vi "Digital Write 1 Channel.vi"(8 "error constant":errorcluster, 9 "Value":bool=TRUE, 10 "Channel":i32, 11 "NI-DAQ.lvclass":refnum<class "NI-DAQ.lvclass">) -> (0 "error IO":errorcluster, 3 "NI-DAQ.lvclass 2":refnum<class "NI-DAQ.lvclass">)   [LabVIEW 2019, in "NI-DAQ.lvclass"]
uses:
  NI-DAQ.lvclass
  NI-DAQ.lvclass/NI-DAQ.ctl
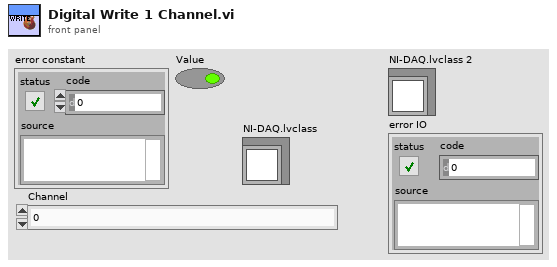
[diagram p1: front panel]
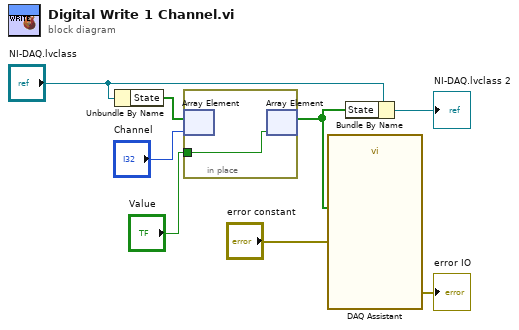
[diagram p0: block diagram]
diagram:
  n1 = Unbundle By Name("NI-DAQ.lvclass") -> ("State"=w4:bool[])
  n2 = in-place {
    in-place-border: "Value" -> [w9]
    n3 = in-place-array #1(w4, "Channel") -> ()  [unwired: 1 out]
    n4 = in-place-array #1(w9) -> (w3:bool[])  [unwired: 1 out]
  }
  n5 = call "DAQ Assistant"("data"=w3, "error in"="error constant") -> ("error out"=→"error IO":errorcluster)  [unwired: 16 in, 1 out]
  n6 = Bundle By Name(cluster="NI-DAQ.lvclass", "State"=w3) -> (→"NI-DAQ.lvclass 2":refnum<class "NI-DAQ.lvclass">)
